vi "Compose LabVIEW Object - Error Input - Returns Same Error.vi"() -> ()   [LabVIEW 2017, in "Composition.Tests.lvlib"]
uses:
  Composition.Tests.lvlib
  c53c5236-6a32-4dca-880e-4ad1106e00ac.vi
  Composition/Get ClassName From Flattened Object.vi
  <vilib>/Utility/error.llb/Error Cluster From Error Code.vi
  <vilib>/Utility/LVClass/Qualified Name Array To Single String.vi
  <vilib>/ErrorRing/Error Ring.xnode
  <vilib>/addons/_JKI Toolkits/Caraya/classes/Assert/Assert.lvclass
  <vilib>/addons/_JKI Toolkits/Caraya/classes/Test/Test.lvclass
panel:
  out "error out":errorcluster
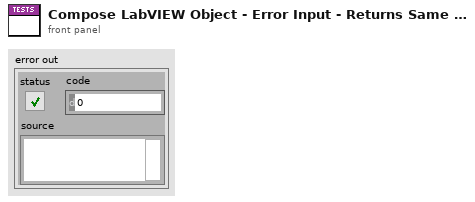
[diagram p1: front panel]
types:
  T1 = cluster{"Major":u16, "Minor":u16, "Fix":u16, "Build":u16}[]
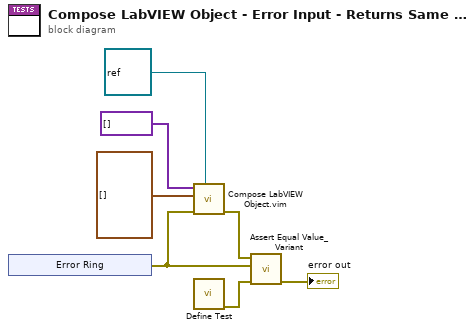
[diagram p0: block diagram]
diagram:
  n1 = xnode "Error Ring"() -> ("error out"=w1:errorcluster)
  n2 = call "Compose LabVIEW Object.vim"("Type"=refnum<class> refnum ("LabVIEW Object"), "error in (no error)"=w1, "Library Versions"=T1 [], "Private Data Clusters"=variant[] []) -> ("error out"=w3:errorcluster)  [unwired: 6 in, 1 out]
  n3 = call <vilib>:"Define Test.vi"() -> ("error out"=w2:errorcluster)  [unwired: 11 in]
  n4 = call <vilib>:"Assert Equal Value_Variant.vi"("error in (no error)"=w2, "Y"=w1, "X"=w3) -> ("error out"=→"error out":errorcluster)  [unwired: 8 in]
